vi "Capture_Save_Initialize_2.0.vi"(1 "Data":T1={"Camera 1"={"Camera1"="", "Cam 1"=FALSE, "CAM1 Model"=enum."a2A5328-15ucBAS", "Cam1 ID"=0}, "Camera 2"={"Camera2"="", "Cam 2"=FALSE, "CAM2 Model"=enum."a2A5328-15ucBAS", "Cam2 ID"=0}, "Image"={"Camera1_Img"=refnum, "Camera2_Img"=refnum, "Img1_Orig_Disp"=refnum, "Img2_Orig_Disp"=refnum, "Img1_Orig_RGB"=refnum, "Img2_Orig_RGB"=refnum, "Blue_Plane_Extract"=refnum, "Subtracted_Plane"=refnum, "Img1_Binary"=refnum, "Img2_Binary"=refnum, "Crop_Mask"=refnum, "Img1_Save"=refnum, "Img2_Save"=refnum, "Img1_Cali_Full"=refnum, "Img2_Cali_Full"=refnum, "Img1_Cali_Detect"=refnum, "Img2_Cali_Detect"=refnum}, "Ques"={"Cam 1 queue"=refnum, "Cam 2 queue"=refnum, "Cam 1 - save queue"=refnum, "Cam 2 - save queue"=refnum, "Image Process Queue Size"=500, "Image Save Queue Size"=500, "Overload threshold"=500, "Max large object threshold"=0}, "Arduino SRS"={"Pinch-valve"="", "Actuator"=FALSE, "Open(T)/Close(F)"=FALSE, "Arduino Uno"=""}, "Pump"={"Port"="", "Connection"=FALSE, "Pump State"=FALSE, "Pump Model"=enum."XLP6000", "Pump size"=FALSE, "Flush Size"=0, "Dispense Speed"=100, "Command"="", "Pump"=""}, "Camera settings"={"Detection settings"={"Sample size threshold"=500, "Detection Region %"=30.0, "Timeout Sample"=200}, "Lens/camera settings"={"Aperture"=enum."Item 0", "Legacy Cam Attributes"=FALSE, "Max Framerate"=100, "Exposure Time"=1000.0, "Framerate"=15}, "Crop settings"={"Cam1"={"Rectangle 1"={"Left"=0, "Top"=0, "Right"=0, "Bottom"=0, "Rotation"=0.0}, "Camera Orientation 1"="", "Pixel to mm 1"=0.0}, "Cam2"={"Rectangle 2"={"Left"=0, "Top"=0, "Right"=0, "Bottom"=0, "Rotation"=0.0}, "Camera Orientation 2"="", "Pixel to mm 2"=0.0}}}, "Arduino ISS"={"Mega F3"="", "Phase3"=FALSE, "Barcode"="", "Sorting sys."=FALSE, "Initial size"=0.0, "Size Interval"=0.0, "Mun. of containers"=0.0, "Container nr."=0.0, "Arduino Mega"=""}, "Img_Capt"=FALSE, "Empty_Refill"=FALSE, "I don't think is in use"={"Crop"=FALSE, "Light intensity"=100, "Empty start"=1}, "Img_Capt Begin"=FALSE, "Extended setup"={"Location"="Station", "Latitude"="Station", "Longitude"="Station", "Determiner"="Station", "Sex"="Station", "Station"="", "Collection date"=""}, "Main interface"={"Sample Name"="Test Sample", "Operator"="JFR", "Species Name"="", "Other Notes"=""}, "Tap1"=0, "SystemVersion"=0, "System Serial"="", "Flush Insect"=FALSE, "Exit"=FALSE, "Kuvette Full"=FALSE, "Core JKI"={"Current VI Reference"=refnum, "Close Panel on Exit?"=FALSE}, "Calibration"={"Calibration 1"=path "C:/Users/au540322/Desktop/IHS_Project/images/Debris/Debris_0/Debris_0_2019_06_01-23-32-49-686.PNG", "Calibration 2"=path "C:/Users/au540322/Desktop/IHS_Project/images/Debris/Debris_0/Debris_0_2019_06_01-23-32-49-686.PNG", "Detect 1"=path "C:/Users/au540322/Desktop/IHS_Project/images/Debris/Debris_0/Debris_0_2019_06_01-23-32-49-686.PNG", "Detect 2"=path "C:/Users/au540322/Desktop/IHS_Project/images/Debris/Debris_0/Debris_0_2019_06_01-23-32-49-686.PNG"}} {"SystemVersion" items=["Standard", "XL"]; "Tap1" items=["Session Data", "Extended Setup", "Buffer", "Camera", "Dispenser", "Stats", "Connections"]; "I don't think is in use"."Empty start" min=1; "I don't think is in use"."Light intensity" scale=0.0..100.0; "Camera settings"."Crop settings"."Cam2"."Rectangle 2"."Rotation" format="%.2f"; "Camera settings"."Crop settings"."Cam2"."Rectangle 2"."Left" scale=0.0..1024.0; "Camera settings"."Crop settings"."Cam2"."Rectangle 2"."Right" scale=0.0..1024.0; "Camera settings"."Crop settings"."Cam1"."Rectangle 1"."Rotation" format="%.2f"; "Camera settings"."Crop settings"."Cam1"."Rectangle 1"."Left" scale=0.0..1024.0; "Camera settings"."Crop settings"."Cam1"."Rectangle 1"."Right" scale=0.0..1024.0; "Camera settings"."Lens/camera settings"."Framerate" min=1; "Camera settings"."Lens/camera settings"."Max Framerate" min=1; "Camera settings"."Detection settings"."Sample size threshold" min=1; "Pump"."Dispense Speed" min=1; "Pump"."Flush Size" min=0 max=6000 step=100; "Ques"."Overload threshold" min=1; "Ques"."Image Save Queue Size" min=1; "Ques"."Image Process Queue Size" min=1}) -> (0 "output cluster":T1={"Camera 1"={"Camera1"="", "Cam 1"=FALSE, "CAM1 Model"=enum."a2A5328-15ucBAS", "Cam1 ID"=0}, "Camera 2"={"Camera2"="", "Cam 2"=FALSE, "CAM2 Model"=enum."a2A5328-15ucBAS", "Cam2 ID"=0}, "Image"={"Camera1_Img"=refnum, "Camera2_Img"=refnum, "Img1_Orig_Disp"=refnum, "Img2_Orig_Disp"=refnum, "Img1_Orig_RGB"=refnum, "Img2_Orig_RGB"=refnum, "Blue_Plane_Extract"=refnum, "Subtracted_Plane"=refnum, "Img1_Binary"=refnum, "Img2_Binary"=refnum, "Crop_Mask"=refnum, "Img1_Save"=refnum, "Img2_Save"=refnum, "Img1_Cali_Full"=refnum, "Img2_Cali_Full"=refnum, "Img1_Cali_Detect"=refnum, "Img2_Cali_Detect"=refnum}, "Ques"={"Cam 1 queue"=refnum, "Cam 2 queue"=refnum, "Cam 1 - save queue"=refnum, "Cam 2 - save queue"=refnum, "Image Process Queue Size"=500, "Image Save Queue Size"=500, "Overload threshold"=500, "Max large object threshold"=0}, "Arduino SRS"={"Pinch-valve"="", "Actuator"=FALSE, "Open(T)/Close(F)"=FALSE, "Arduino Uno"=""}, "Pump"={"Port"="", "Connection"=FALSE, "Pump State"=FALSE, "Pump Model"=enum."XLP6000", "Pump size"=FALSE, "Flush Size"=0, "Dispense Speed"=100, "Command"="", "Pump"=""}, "Camera settings"={"Detection settings"={"Sample size threshold"=500, "Detection Region %"=30.0, "Timeout Sample"=200}, "Lens/camera settings"={"Aperture"=enum."Item 0", "Legacy Cam Attributes"=FALSE, "Max Framerate"=100, "Exposure Time"=1000.0, "Framerate"=15}, "Crop settings"={"Cam1"={"Rectangle 1"={"Left"=0, "Top"=0, "Right"=0, "Bottom"=0, "Rotation"=0.0}, "Camera Orientation 1"="", "Pixel to mm 1"=0.0}, "Cam2"={"Rectangle 2"={"Left"=0, "Top"=0, "Right"=0, "Bottom"=0, "Rotation"=0.0}, "Camera Orientation 2"="", "Pixel to mm 2"=0.0}}}, "Arduino ISS"={"Mega F3"="", "Phase3"=FALSE, "Barcode"="", "Sorting sys."=FALSE, "Initial size"=0.0, "Size Interval"=0.0, "Mun. of containers"=0.0, "Container nr."=0.0, "Arduino Mega"=""}, "Img_Capt"=FALSE, "Empty_Refill"=FALSE, "I don't think is in use"={"Crop"=FALSE, "Light intensity"=100, "Empty start"=1}, "Img_Capt Begin"=FALSE, "Extended setup"={"Location"="Station", "Latitude"="Station", "Longitude"="Station", "Determiner"="Station", "Sex"="Station", "Station"="", "Collection date"=""}, "Main interface"={"Sample Name"="Test Sample", "Operator"="JFR", "Species Name"="", "Other Notes"=""}, "Tap1"=0, "SystemVersion"=0, "System Serial"="", "Flush Insect"=FALSE, "Exit"=FALSE, "Kuvette Full"=FALSE, "Core JKI"={"Current VI Reference"=refnum, "Close Panel on Exit?"=FALSE}, "Calibration"={"Calibration 1"=path "C:/Users/au540322/Desktop/IHS_Project/images/Debris/Debris_0/Debris_0_2019_06_01-23-32-49-686.PNG", "Calibration 2"=path "C:/Users/au540322/Desktop/IHS_Project/images/Debris/Debris_0/Debris_0_2019_06_01-23-32-49-686.PNG", "Detect 1"=path "C:/Users/au540322/Desktop/IHS_Project/images/Debris/Debris_0/Debris_0_2019_06_01-23-32-49-686.PNG", "Detect 2"=path "C:/Users/au540322/Desktop/IHS_Project/images/Debris/Debris_0/Debris_0_2019_06_01-23-32-49-686.PNG"}} {"SystemVersion" items=["Standard", "XL"]; "Tap1" items=["Session Data", "Extended Setup", "Buffer", "Camera", "Dispenser", "Stats", "Connections"]; "I don't think is in use"."Empty start" min=1; "I don't think is in use"."Light intensity" scale=0.0..100.0; "Camera settings"."Crop settings"."Cam2"."Rectangle 2"."Rotation" format="%.2f"; "Camera settings"."Crop settings"."Cam2"."Rectangle 2"."Left" scale=0.0..1024.0; "Camera settings"."Crop settings"."Cam2"."Rectangle 2"."Right" scale=0.0..1024.0; "Camera settings"."Crop settings"."Cam1"."Rectangle 1"."Rotation" format="%.2f"; "Camera settings"."Crop settings"."Cam1"."Rectangle 1"."Left" scale=0.0..1024.0; "Camera settings"."Crop settings"."Cam1"."Rectangle 1"."Right" scale=0.0..1024.0; "Camera settings"."Lens/camera settings"."Framerate" min=1; "Camera settings"."Lens/camera settings"."Max Framerate" min=1; "Camera settings"."Detection settings"."Sample size threshold" min=1; "Pump"."Dispense Speed" min=1; "Pump"."Flush Size" min=0 max=6000 step=100; "Ques"."Overload threshold" min=1; "Ques"."Image Save Queue Size" min=1; "Ques"."Image Process Queue Size" min=1})   [LabVIEW 2024]
uses:
  controls/Data_JKI.ctl
  <vilib>/userDefined/High Color/IMAQdx.ctl
  <vilib>/vision/Image Controls.llb/IMAQ Image.ctl
  <vilib>/vision/driver/IMAQdx.llb/IMAQdx Acquisition Mode.ctl
  <vilib>/vision/driver/NI_Vision_Acquisition_Software.lvlib
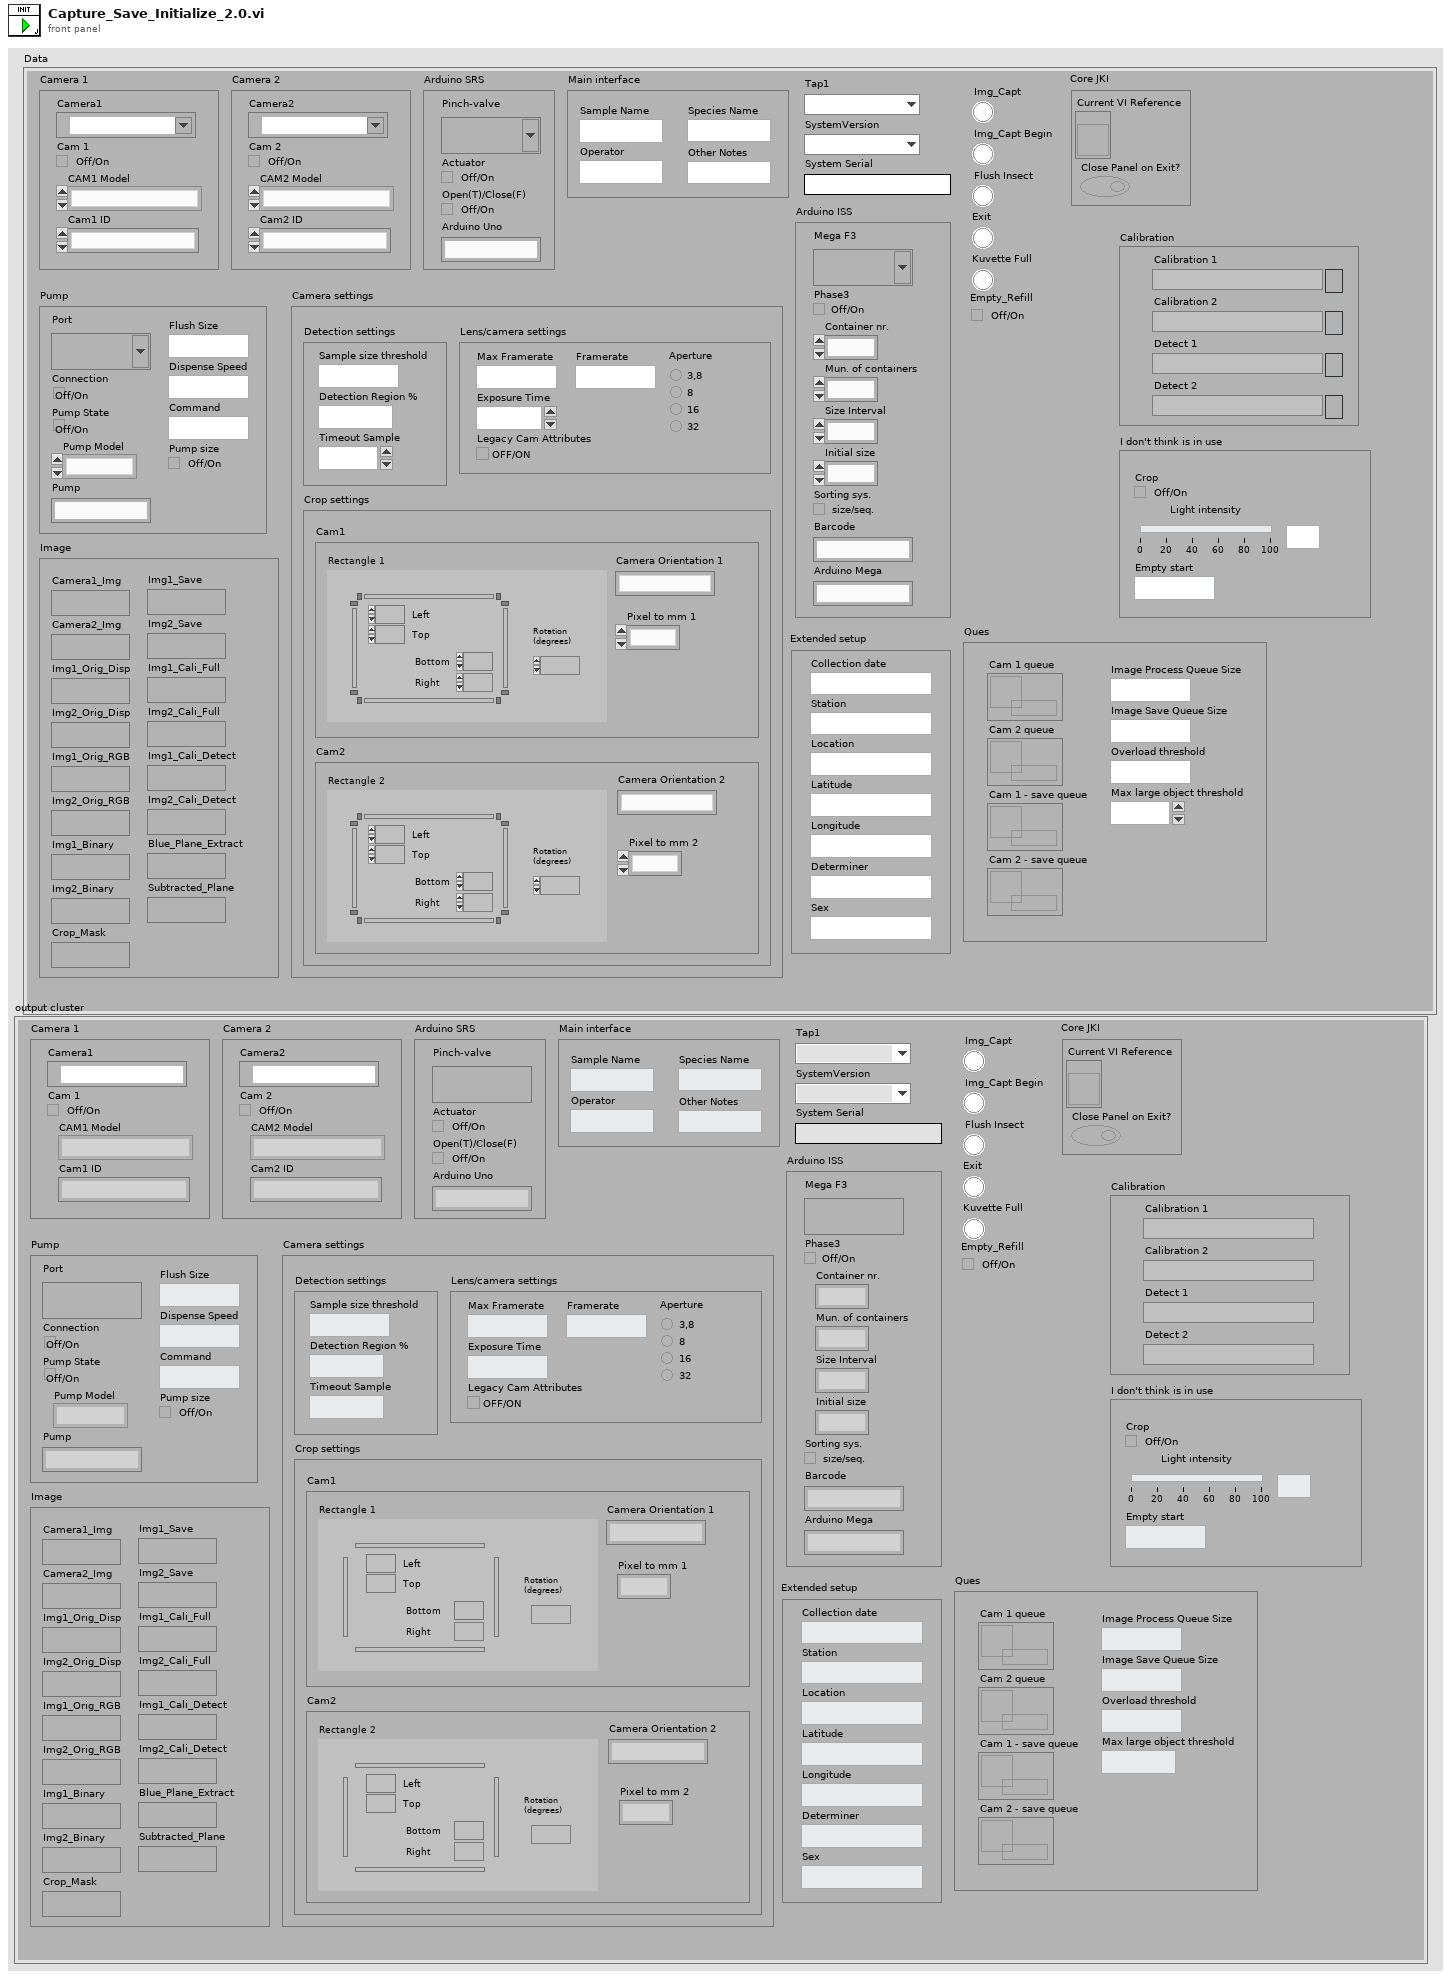
[diagram p1: front panel]
types:
  T1 = typedef "Data_JKI.ctl" = cluster{"Camera 1":cluster{"Camera1":T2, "Cam 1":bool, "CAM1 Model":enum16{"a2A5328-15ucBAS", "acA1920-155uc"}, "Cam1 ID":i32}, "Camera 2":cluster{"Camera2":T2, "Cam 2":bool, "CAM2 Model":enum16{"a2A5328-15ucBAS", "acA1920-155uc"}, "Cam2 ID":i32}, "Image":cluster{"Camera1_Img":T3, "Camera2_Img":T3, "Img1_Orig_Disp":T3, "Img2_Orig_Disp":T3, "Img1_Orig_RGB":T3, "Img2_Orig_RGB":T3, "Blue_Plane_Extract":T3, "Subtracted_Plane":T3, "Img1_Binary":T3, "Img2_Binary":T3, "Crop_Mask":T3, "Img1_Save":T3, "Img2_Save":T3, "Img1_Cali_Full":T3, "Img2_Cali_Full":T3, "Img1_Cali_Detect":T3, "Img2_Cali_Detect":T3}, "Ques":cluster{"Cam 1 queue":refnum<queue>, "Cam 2 queue":refnum<queue>, "Cam 1 - save queue":refnum<queue>, "Cam 2 - save queue":refnum<queue>, "Image Process Queue Size":i32, "Image Save Queue Size":i32, "Overload threshold":i32, "Max large object threshold":i32}, "Arduino SRS":cluster{"Pinch-valve":refnum<visa-resource-name>, "Actuator":bool, "Open(T)/Close(F)":bool, "Arduino Uno":string}, "Pump":cluster{"Port":refnum<visa-resource-name>, "Connection":bool, "Pump State":bool, "Pump Model":enum16{"XLP6000", "XL1000"}, "Pump size":bool, "Flush Size":i32, "Dispense Speed":i32, "Command":string, "Pump":string}, "Camera settings":cluster{"Detection settings":cluster{"Sample size threshold":i32, "Detection Region %":dbl, "Timeout Sample":i32}, "Lens/camera settings":cluster{"Aperture":enum32{"Item 0", "Item 1", "Item 2", "Item 3"}, "Legacy Cam Attributes":bool, "Max Framerate":i32, "Exposure Time":dbl, "Framerate":i32}, "Crop settings":cluster{"Cam1":cluster{"Rectangle 1":T4, "Camera Orientation 1":string, "Pixel to mm 1":dbl}, "Cam2":cluster{"Rectangle 2":T4, "Camera Orientation 2":string, "Pixel to mm 2":dbl}}}, "Arduino ISS":cluster{"Mega F3":refnum<visa-resource-name>, "Phase3":bool, "Barcode":string, "Sorting sys.":bool, "Initial size":dbl, "Size Interval":dbl, "Mun. of containers":dbl, "Container nr.":dbl, "Arduino Mega":string}, "Img_Capt":bool, "Empty_Refill":bool, "I don't think is in use":cluster{"Crop":bool, "Light intensity":i32, "Empty start":u32}, "Img_Capt Begin":bool, "Extended setup":cluster{"Location":string, "Latitude":string, "Longitude":string, "Determiner":string, "Sex":string, "Station":string, "Collection date":string}, "Main interface":cluster{"Sample Name":string, "Operator":string, "Species Name":string, "Other Notes":string}, "Tap1":u16, "SystemVersion":u16, "System Serial":string, "Flush Insect":bool, "Exit":bool, "Kuvette Full":bool, "Core JKI":cluster{"Current VI Reference":refnum<vi>, "Close Panel on Exit?":bool}, "Calibration":cluster{"Calibration 1":path, "Calibration 2":path, "Detect 1":path, "Detect 2":path}}
  T2 = typedef "IMAQdx.ctl" = refnum<k21>
  T3 = typedef "IMAQ Image.ctl" = refnum<image>
  T4 = typedef "IMAQ Rectangle" = cluster{"Left":i32, "Top":i32, "Right":i32, "Bottom":i32, "Rotation":dbl}
  T5 = typedef "Image Type" = u32
  T6 = cluster{"Timestamp":string, "Image Pixels (U32)":u32[][], "Prev. sample":i32, "Sample Data":dbl[], "output cluster":cluster{"Global Rectangle":i32[], "Contours":cluster{"ID":enum32{"External", "Internal"}, "Type":u32, "Coordinates":i32[]}[]}}
  T7 = cluster{"Image Pixels (U32)":u32[][], "Detect Movement":bool, string}
  T8 = typedef "NI_Vision_Acquisition_Software.lvlib/IMAQdx Acquisition Mode.ctl" = enum32{"One Shot", "Continuous"}
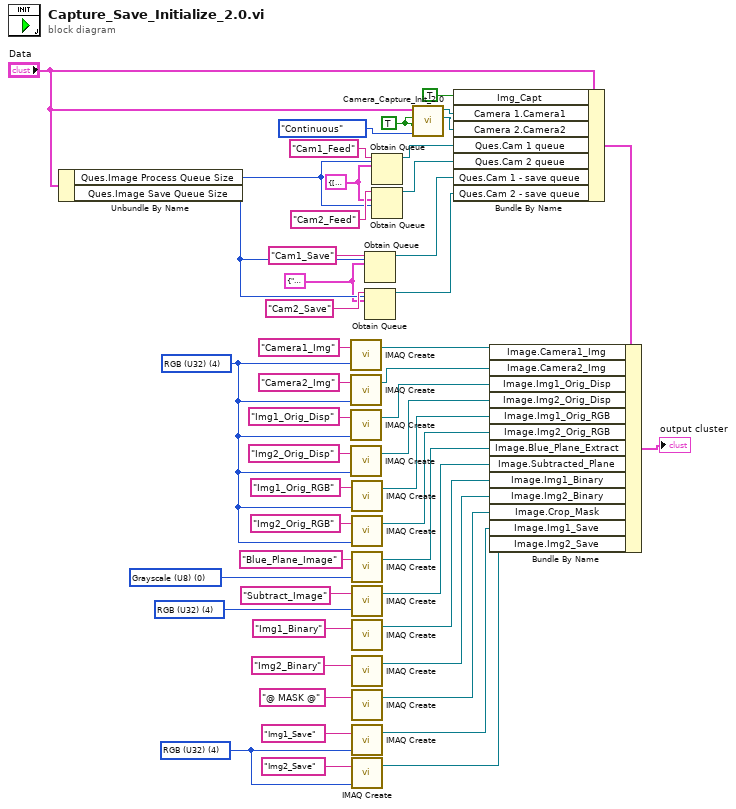
[diagram p0: block diagram]
diagram:
  w7 = T5 0 items=["Grayscale (U8)", "Grayscale (I16)", "Grayscale (SGL)", "Complex (CSG)", "RGB (U32)", "HSL (U32)", "RGB (U64)", "Grayscale (U16)"] ("Image Type")
  w8 = T5 4 items=["Grayscale (U8)", "Grayscale (I16)", "Grayscale (SGL)", "Complex (CSG)", "RGB (U32)", "HSL (U32)", "RGB (U64)", "Grayscale (U16)"] ("Image Type")
  w9 = T6 {"Timestamp"="", "Image Pixels (U32)"=[], "Prev. sample"=0, "Sample Data"=[], "output cluster"={"Global Rectangle"=[], "Contours"=[]}} ("output cluster")
  w10 = T7 {"Image Pixels (U32)"=[], "Detect Movement"=FALSE, ""} ("output cluster")
  w26 = T5 4 items=["Grayscale (U8)", "Grayscale (I16)", "Grayscale (SGL)", "Complex (CSG)", "RGB (U32)", "HSL (U32)", "RGB (U64)", "Grayscale (U16)"] ("Image Type")
  w11 = T5 4 items=["Grayscale (U8)", "Grayscale (I16)", "Grayscale (SGL)", "Complex (CSG)", "RGB (U32)", "HSL (U32)", "RGB (U64)", "Grayscale (U16)"] ("Image Type")
  w2 = TRUE ("Crop?")
  n1 = Unbundle By Name("Data") -> ("Ques.Image Process Queue Size"=w39:i32, "Ques.Image Save Queue Size"=w29:i32)
  n2 = call "IMAQ Create"("Image Name"="Camera1_Img", "Image Type"=w11) -> ("New Image"=w25:T3)  [unwired: 3 in, 1 out]
  n3 = call "IMAQ Create"("Image Name"="Camera2_Img", "Image Type"=w11) -> ("New Image"=w24:T3)  [unwired: 3 in, 1 out]
  n4 = call "IMAQ Create"("Image Name"="Img1_Orig_Disp", "Image Type"=w11) -> ("New Image"=w23:T3)  [unwired: 2 in, 2 out]
  n5 = call "IMAQ Create"("Image Name"="Img2_Orig_Disp", "Image Type"=w11) -> ("New Image"=w22:T3)  [unwired: 2 in, 2 out]
  n6 = call "IMAQ Create"("Image Name"="Img1_Orig_RGB", "Image Type"=w11) -> ("New Image"=w21:T3)  [unwired: 2 in, 2 out]
  n7 = call "IMAQ Create"("Image Name"="Img2_Orig_RGB", "Image Type"=w11) -> ("New Image"=w20:T3)  [unwired: 2 in, 2 out]
  n8 = call "IMAQ Create"("Image Name"="Blue_Plane_Image", "Image Type"=w7) -> ("New Image"=w19:T3)  [unwired: 2 in, 2 out]
  n9 = call "IMAQ Create"("Image Name"="Subtract_Image", "Image Type"=w8) -> ("New Image"=w18:T3)  [unwired: 2 in, 2 out]
  n10 = call "IMAQ Create"("Image Name"="Img1_Binary") -> ("New Image"=w17:T3)  [unwired: 3 in, 2 out]
  n11 = call "IMAQ Create"("Image Name"="Img2_Binary") -> ("New Image"=w16:T3)  [unwired: 3 in, 2 out]
  n12 = call "IMAQ Create"("Image Name"="@ MASK @") -> ("New Image"=w15:T3)  [unwired: 3 in, 2 out]
  n13 = call "IMAQ Create"("Image Name"="Img1_Save", "Image Type"=w26) -> ("New Image"=w14:T3)  [unwired: 2 in, 2 out]
  n14 = call "IMAQ Create"("Image Name"="Img2_Save", "Image Type"=w26) -> ("New Image"=w13:T3)  [unwired: 2 in, 2 out]
  n15 = Obtain Queue(max queue size (-1, unlimited)=w29, name (unnamed)="Cam1_Save", element data type=w9) -> (queue out=w33:refnum<queue>)  [unwired: 2 in, 2 out]
  n16 = Obtain Queue(max queue size (-1, unlimited)=w29, name (unnamed)="Cam2_Save", element data type=w9) -> (queue out=w32:refnum<queue>)  [unwired: 2 in, 2 out]
  n17 = Obtain Queue(max queue size (-1, unlimited)=w39, name (unnamed)="Cam1_Feed", element data type=w10) -> (queue out=w45:refnum<queue>)  [unwired: 2 in, 2 out]
  n18 = Obtain Queue(max queue size (-1, unlimited)=w39, name (unnamed)="Cam2_Feed", element data type=w10) -> (queue out=w44:refnum<queue>)  [unwired: 2 in, 2 out]
  n19 = call "Camera_Capture_Init_2.0.vi"("Continuous?"=IMAQdx_Acquisition_Mode."Continuous", "Detect Movement"=w2, "Crop?"=w2, "Data"="Data") -> ("Camera2"=w3:T2, "Camera1"=w4:T2)  [unwired: 6 in]
  n20 = Bundle By Name(cluster="Data", "Img_Capt"=TRUE ("Image_Capture"), "Camera 1.Camera1"=w4, "Camera 2.Camera2"=w3, "Ques.Cam 1 queue"=w45, "Ques.Cam 2 queue"=w44, "Ques.Cam 1 - save queue"=w33, "Ques.Cam 2 - save queue"=w32) -> (w28:T1)
  n21 = Bundle By Name(cluster=w28, "Image.Camera1_Img"=w25, "Image.Camera2_Img"=w24, "Image.Img1_Orig_Disp"=w23, "Image.Img2_Orig_Disp"=w22, "Image.Img1_Orig_RGB"=w21, "Image.Img2_Orig_RGB"=w20, "Image.Blue_Plane_Extract"=w19, "Image.Subtracted_Plane"=w18, "Image.Img1_Binary"=w17, "Image.Img2_Binary"=w16, "Image.Crop_Mask"=w15, "Image.Img1_Save"=w14, "Image.Img2_Save"=w13) -> (→"output cluster":T1)
